vi "CreateBuffer.vi"(8 "error in (no error)":errorcluster, 9 "Buffer size":i32, 10 "Data type":T1(ring)=enum."I16") -> (0 "error out":errorcluster, 2 "Pointer and BufferSize":u64[](array[numeric]))   [LabVIEW 2020]
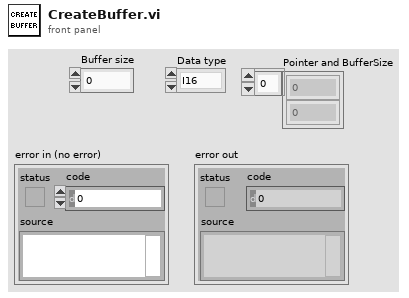
[diagram p1: front panel]
types:
  T1 = enum16{"U8", "I8", "U16", "I16", "U32", "I32", "U64", "I64"}
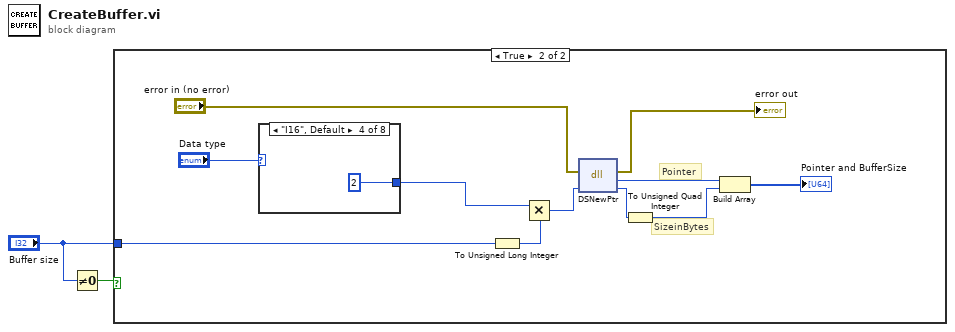
[diagram p0: block diagram]
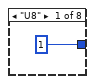
[diagram p3: hidden frame]
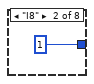
[diagram p4: hidden frame]
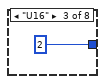
[diagram p5: hidden frame]
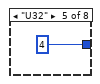
[diagram p6: hidden frame]
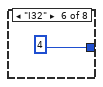
[diagram p7: hidden frame]
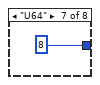
[diagram p8: hidden frame]
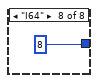
[diagram p9: hidden frame]
diagram:
  n1 = Not Equal To 0?(x="Buffer size") -> (x != 0?=w1:bool)
  n2 = case shown="True" w1 {
    tunnel: "Buffer size" -> [_ w6]
    frame False {
    }
    frame True {
      # "Pointer"
      # "SizeinBytes"
      n3 = case shown="\"I16\", Default" "Data type" {
        tunnel: [u32 1 ("element") u32 1 ("element") u32 2 ("element") u32 2 ("element") u32 4 ("element") u32 4 ("element") u32 8 ("element") u32 8 ("element")] -> w3
        frame "U8" {
        }
        frame "I8" {
        }
        frame "U16" {
        }
        frame "I16", Default {
        }
        frame "U32" {
        }
        frame "I32" {
        }
        frame "U64" {
        }
        frame "I64" {
        }
      }
      n4 = To Unsigned Long Integer(number=w6) -> (unsigned 32bit integer=w9:u32)
      n5 = Multiply(x=w3, y=w9) -> (x*y=w13:u32)
      n6 = dll-call lib="LabVIEW" fn="DSNewPtr"(error in="error in (no error)", "Size"=w13) -> (error out=→"error out":errorcluster, "Pointer"=w12:u32, "Size"=w11:u32)  [unwired: 2 in, 1 out]
      n7 = To Unsigned Quad Integer(1:w11) -> (0:w10:u64)
      n8 = Build Array(w12, w10) -> (→"Pointer and BufferSize":u64[])
    }
  }
